vi "GDSLvClass_GetClassMethod.vi"(0 "Class Refnum In":refnum<vi>, 1 "VINames":string[](array[string]), 5 "error in (no error)":errorcluster) -> (12 "AllClassFiles":path[](array[path]), 14 "Class Refnum Out":refnum<vi>, 15 "ViPaths":path[](array[path]), 19 "error out":errorcluster)   [LabVIEW 2012]
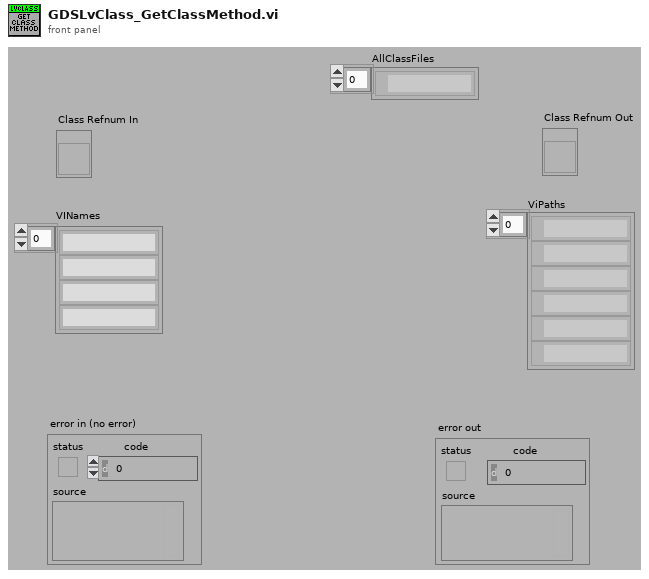
[diagram p1: front panel]
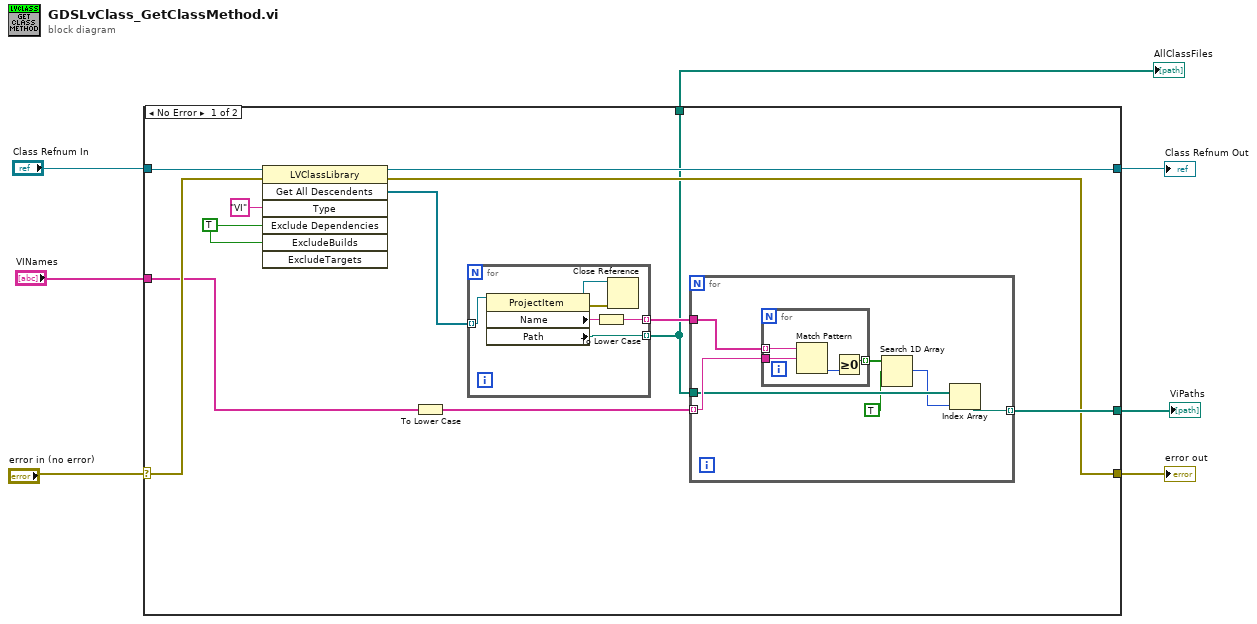
[diagram p0: block diagram]
diagram:
  n1 = case shown="No Error" "error in (no error)" {
    selector: "error in (no error)" -> [w18 w38]
    tunnel: [w11 w38] -> w6
    tunnel: "Class Refnum In" -> [w19 w37]
    tunnel: [w10 w37] -> w4
    tunnel: "VINames" -> [w15 _]
    tunnel: [w12 _] -> w2
    tunnel: [w9 _] -> w1
    frame No Error {
      w8 = TRUE ("ExcludeDependencies")
      n2 = invoke class="LVClassLibrary" method="Get All Descendents"(reference=w19, error in=w18, "Type"="VI", "Exclude Dependencies"=w8, "ExcludeBuilds"=w8) -> (reference out=w10:refnum<vi>, error out=w11:errorcluster, "All Descendents"=w16:refnum<vi>[])  [unwired: 2 in, 4 out]
      n3 = To Lower Case(string=w15) -> (all lower case string=w13:string[])
      n4 = for {
        tunnel: w16 -> [w36] mode=indexing
        tunnel: [w34] -> w14 mode=indexing
        tunnel: [w33] -> w9 mode=indexing
        n5 = property class="ProjectItem"(reference=w36) -> (reference out=w31:refnum<vi>, error out=w32:errorcluster, "Name"=w35:string, "Path"=w33:path)  [unwired: 1 in]
        n6 = To Lower Case(string=w35) -> (all lower case string=w34:string)
        n7 = Close Reference(reference=w31, error in (no error)=w32) -> ()  [unwired: 1 out]
      }
      n8 = for {
        tunnel: w14 -> [w26]
        tunnel: w13 -> [w25] mode=indexing
        tunnel: w9 -> [w24]
        tunnel: [w23] -> w12 mode=indexing
        n9 = for {
          tunnel: w26 -> [w30] mode=indexing
          tunnel: w25 -> [w29]
          tunnel: [w27] -> w22 mode=indexing
          n10 = Match Pattern(string=w30, regular expression=w29) -> (offset past match=w28:i32)  [unwired: 1 in, 3 out]
          n11 = Greater Or Equal To 0?(x=w28) -> (x >= 0?=w27:bool)
        }
        n12 = Search 1D Array(1D array=w22, element=TRUE) -> (index of element=w20:i32)  [unwired: 1 in]
        n13 = Index Array(array=w24, index=w20) -> (element=w23:path)
      }
    }
    frame Error {
    }
  }
  "Class Refnum Out" <- w4
  "error out" <- w6
  "ViPaths" <- w2
  "AllClassFiles" <- w1
